vi "_Prepare Run Data.vi"(8 "error in (no error)":errorcluster) -> (0 "error out":errorcluster, 1 "AcqMethod":T1[](array[typedef]) {"ScanType" format="%#.6g"; "Mass Range"."Res" items=["High/High", "Medium/Medium", "Low/Low", "High/Medium", "High/Low", "Medium/High", "Medium/Low", "Low/High", "Low/Medium"]}, 3 "Scans":i32=5, 4 "Total Time (mS)":dbl, 5 "Stop Mass (amu)":dbl=200.0, 6 "Step Size (amu)":dbl=0.1 min=0.01, 7 "Start Mass (amu)":dbl=100.0)   [LabVIEW 2012]
uses:
  Type/_XML Expt.ctl
  Type/_XML Lens.ctl
  Type/_Mass Range Property.ctl
  Type/_Mass Range Parameters.ctl
  Type/_RT Res Type.ctl
  _Global Configuration.vi
panel:
  # "(# of Expts) X (# of MassRanges)"
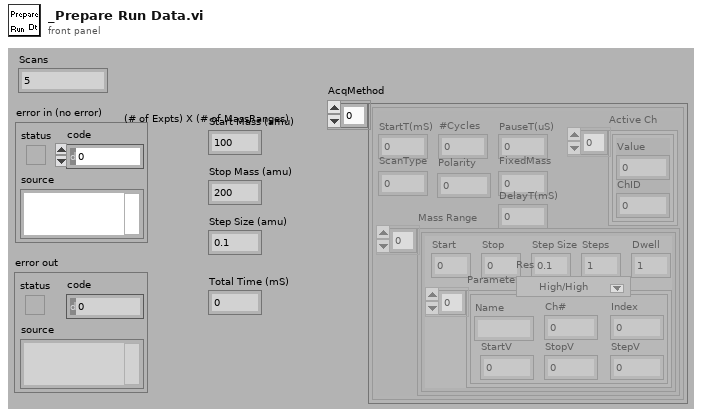
[diagram p1: front panel]
types:
  T1 = typedef "_XML Expt.ctl" = cluster{"StartT(mS)":i32, "#Cycles":i32, "PauseT(uS)":i32, "ScanType":i32, "Polarity":u8, "FixedMass":dbl, "DelayT(mS)":i32, "Active Ch":T2[], "Mass Range":T3[]}
  T2 = typedef "_XML Lens.ctl" = cluster{"Value":dbl, "ChID":u8}
  T3 = typedef "_Mass Range Property.ctl" = cluster{"Start":dbl, "Stop":dbl, "Step Size":dbl, "Steps":i32, "Dwell":dbl, "Parameters":T4[], "Res":T5}
  T4 = typedef "_Mass Range Parameters.ctl" = cluster{"Name":string, "Ch#":u8, "StartV":dbl, "StopV":dbl, "StepV":dbl, "Index":u8}
  T5 = typedef "_RT Res Type.ctl" = u16
  T6 = typedef "_Run Module.ctl" = u16
  T7 = typedef "_Ramp Parameter.ctl" = cluster{"Name":string, "Channel":u8, "Offset":dbl, "Slope":dbl, "Count 1":dbl, "Count 2":dbl, "Time 1":dbl, "Time 2":dbl, "Scans":i32, "Step Size":dbl}
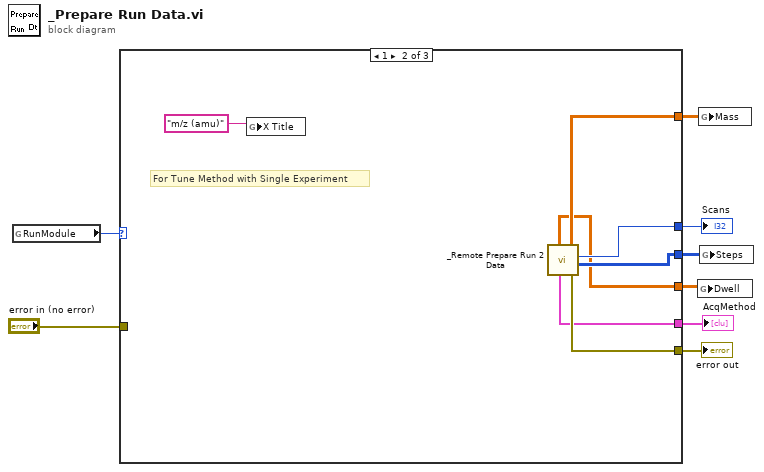
[diagram p0: block diagram]
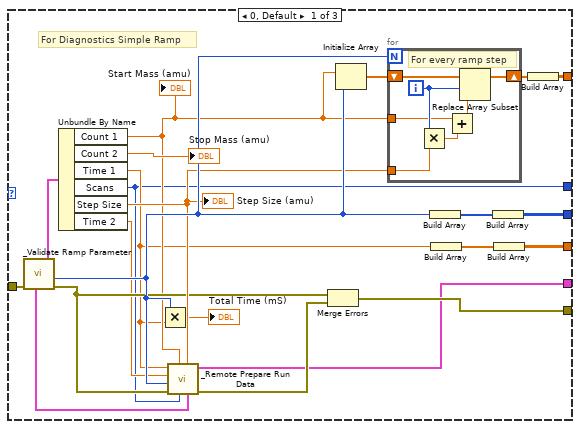
[diagram p2: hidden frame]
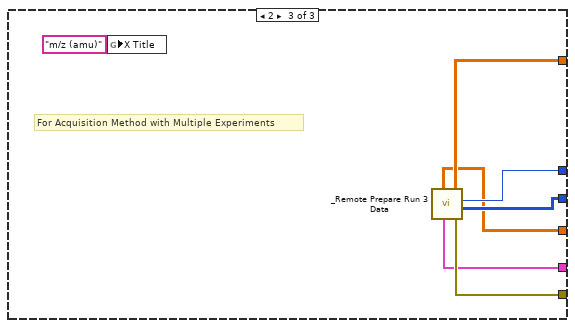
[diagram p3: hidden frame]
diagram:
  n1 = global read "_Global Configuration.vi" "RunModule"() -> (w4:T6)
  n2 = case shown="1" w4 {
    tunnel: [w16 w42 w49] -> w8
    tunnel: "error in (no error)" -> [w28 _ _]
    tunnel: [w14 w44 w51] -> w3
    tunnel: [w22 w40 w46] -> w6
    tunnel: [w10 w43 w50] -> w5
    tunnel: [w11 w41 w47] -> w2
    tunnel: [w9 w39 w45] -> w1
    frame 0, Default {
      # "For Diagnostics Simple Ramp"
      n3 = call "_Validate Ramp Parameter.vi"("error in (no error)"=w28) -> ("error out"=w20:errorcluster, "Steps"=w25:i32, "Primary Parameter"=w27:T7, "Ramp Parameters"=w24:T7[])  [unwired: 4 out]
      n4 = Unbundle By Name(w27) -> ("Count 1"=w19:dbl, "Count 2"=→"Stop Mass (amu)":dbl, "Time 1"=w12:dbl, "Scans"=w10:i32, "Step Size"=w21:dbl, "Time 2"=w17:dbl)
      "Start Mass (amu)" <- w19
      "Step Size (amu)" <- w21
      n5 = Multiply(x=w25, y=w12) -> (x*y=→"Total Time (mS)":dbl)
      n6 = call "_Remote Prepare Run Data.vi"("Ramp Parameters"=w24, "StepMass"=w21, "# of Cycles"=w10, "StartMass"=w19, "error in"=w20, "Steps"=w25, "Pause (ms)"=w17, "Dwell (ms)"=w12) -> ("error out"=w23:errorcluster, "AcqMethod"=w9:T1[])  [unwired: 2 out]
      n7 = Merge Errors(w20, w23) -> (w22:errorcluster)
      n8 = Initialize Array(w19, w25) -> (w30:dbl[])
      n9 = for {
        N: w25 -> [_]
        tunnel: w21 -> [w34]
        shift-right: [w36] -> w29
        shift-left: w30 -> [w37]
        tunnel: w19 -> [w32]
        i -> [w35]
        # "For every ramp step"
        n10 = Multiply(x=w35, y=w34) -> (x*y=w33:dbl)
        n11 = Add(x=w32, y=w33) -> (x+y=w31:dbl)
        n12 = Replace Array Subset(array=w37, new element=w31, index=w35) -> (w36:dbl[])
      }
      n13 = Build Array(w25) -> (w15:i32[])
      n14 = Build Array(w12) -> (w13:dbl[])
      n15 = Build Array(w15) -> (w14:i32[][])
      n16 = Build Array(w13) -> (w11:dbl[][])
      n17 = Build Array(w29) -> (w16:dbl[][])
    }
    frame 1 {
      # "For Tune Method with Single Experiment"
      n18 = global write "_Global Configuration.vi" "X Title"("m/z (amu)" ("X Title")) -> ()
      n19 = call "_Remote Prepare Run 2 Data.vi"() -> ("error out"=w40:errorcluster, "Steps"=w44:i32[][], "Scans"=w43:i32, "Mass"=w42:dbl[][], "AcqMethod"=w39:T1[], "Dwell"=w41:dbl[][])  [unwired: 1 in, 3 out]
    }
    frame 2 {
      # "For Acquisition Method with Multiple Experiments"
      n20 = global write "_Global Configuration.vi" "X Title"("m/z (amu)" ("X Title")) -> ()
      n21 = call "_Remote Prepare Run 3 Data.vi"() -> ("error out"=w46:errorcluster, "Steps"=w51:i32[][], "Scans"=w50:i32, "Mass"=w49:dbl[][], "AcqMethod"=w45:T1[], "Dwell"=w47:dbl[][])  [unwired: 1 in, 3 out]
    }
  }
  "Scans" <- w5
  "error out" <- w6
  "AcqMethod" <- w1
  n22 = global write "_Global Configuration.vi" "Dwell"(w2) -> ()
  n23 = global write "_Global Configuration.vi" "Mass"(w8) -> ()
  n24 = global write "_Global Configuration.vi" "Steps"(w3) -> ()
